vi "MAIN_HGB2_rev01.vi"() -> ()   [LabVIEW 2016]
uses:
  Producer_Case_Structure.ctl
  <vilib>/Utility/error.llb/DialogType.ctl
  <vilib>/express/express analysis/Spectral/XNode/ExpressSpectralMeasurementsBlockNode.xnode
  <vilib>/express/express analysis/Spectral/Block/exnSpectralBlock spectral measurements RMS poly.vi
  <vilib>/express/express analysis/Spectral/Block/exnSpectralBlock spectral measurements RMS array WFM.vi
  <vilib>/DAQmx/write.llb/DAQmx Write (Analog 1D DBL NChan 1Samp).vi
panel:
  out "Compressor Speed":dbl
  out "Run Loop Counter":dbl=67.0
  in  "Speed Setpoint":dbl
  in  "Operator Notes":string
  in  "Dummy Variable":dbl
  in  "Record Data":bool
  in  "Sample Rate [S/s]":dbl=10.0
  in  "file path":path=path "S:/002 - Projects/200804 AECSSB/6-Testing/TDMS Data/raw/080421-1"
  in  "Stop":bool=TRUE
  in  "Tab Control":T1(tab)=enum."Pressure & Temperature"
  out "System Temperatures":waveform(dbl)[](graph)=[{"t0"=timestamp(3710938237.209422 s since 1904-01-01), "dt"=0.1, "Y"=[25.06420596580779], "attributes"=variant("NI_ChannelName"=variant(string "T_dis"), "NI_UnitDescription"=variant(string "Deg C"))}, {"t0"=timestamp(3710938237.209422 s since 1904-01-01), "dt"=0.1, "Y"=[24.5131871952291], "attributes"=variant("NI_ChannelName"=variant(string "T_liq_mix"), "NI_UnitDescription"=variant(string "Deg C"))}, {"t0"=timestamp(3710938237.209422 s since 1904-01-01), "dt"=0.1, "Y"=[24.404692160048143], "attributes"=variant("NI_ChannelName"=variant(string "T_gas_mix"), "NI_UnitDescription"=variant(string "Deg C"))}, {"t0"=timestamp(3710938237.209422 s since 1904-01-01), "dt"=0.1, "Y"=[24.9517211018332], "attributes"=variant("NI_ChannelName"=variant(string "T_wf_cond_out"), "NI_UnitDescription"=variant(string "Deg C"))}, {"t0"=timestamp(3710938237.209422 s since 1904-01-01), "dt"=0.1, "Y"=[24.75846841874906], "attributes"=variant("NI_ChannelName"=variant(string "T_cf_in"), "NI_UnitDescription"=variant(string "Deg C"))}]
  out "Power Constituents":waveform(dbl)[](graph)=[{"t0"=timestamp(3710938237.209422 s since 1904-01-01), "dt"=0.1, "Y"=[-0.0627204059992863], "attributes"=variant("NI_ChannelName"=variant(string "Voltage"))}, {"t0"=timestamp(3710938237.209422 s since 1904-01-01), "dt"=0.1, "Y"=[-0.029340257114334634], "attributes"=variant("NI_ChannelName"=variant(string "Frequency"))}, {"t0"=timestamp(3710938237.0104485 s since 1904-01-01), "dt"=0.1, "Y"=[], "attributes"=variant("NI_ChannelName"=variant(string "Torque"))}]
  out "System Pressures":waveform(dbl)[](graph)=[{"t0"=timestamp(3710938237.209422 s since 1904-01-01), "dt"=0.1, "Y"=[653.0149804276925], "attributes"=variant("NI_ChannelName"=variant(string "P_comp_suc"))}, {"t0"=timestamp(3710938237.209422 s since 1904-01-01), "dt"=0.1, "Y"=[652.9848572024544], "attributes"=variant("NI_ChannelName"=variant(string "P_comp_dis"))}, {"t0"=timestamp(3710938237.209422 s since 1904-01-01), "dt"=0.1, "Y"=[653.0856354357659], "attributes"=variant("NI_ChannelName"=variant(string "P_comp_int"))}]
  out "Mass Flow":waveform(dbl)(graph)={"t0"=timestamp(3710938237.209422 s since 1904-01-01), "dt"=0.1, "Y"=[-2.0362630357040334e-05], "attributes"=variant("NI_ChannelName"=variant(string "m_dot_wf"))}
  out "Raw Acceleration":waveform(dbl)[](graph)
  out "Accel. Spectrum":cluster{"f0":dbl, "df":dbl, "magnitude":dbl[]}[](graph)
  in  "?":path=path "C:/Users/ASITest/Desktop/REFPROP"
  in  "Working Fluid":string="R134A.FLD"
  out "Sound":waveform(dbl)(graph)
  in  "Range":enum16{"40-70 dB", "auto", "60-90 dB"}(ring)
  in  "Ambient Noise [dB]":dbl=74.0
  # "Stop VI"
  # "Air Squared Hot Gas Bypass Test Stand"
  # "Point to where REFPROP is..."
  # "Registar Index of Calc Characteristics"
  # "INPUT NEEDED"
  # "0 = No\n1 = Yes"
  # "0 = No\n1 = Yes"
  # "UNITS:\nkg/s\nC\nRPM\nkPa\nV\nA"
  # "... where is the sensor in the initialization indexing?"
  # "Must have sound meter set up to manual range:\n1. click 'RNG' button on the meter \n2. the value displayed under 'SPL' on the display is the min of the range\n3. ensure the meter is on 'FAST' mode by clicking 'F/S', 'FAST' will be read on display\n4. use the A/C to select 'A' mode displayed on meter\n5. BEFORE INITIALIZING - set ambient noise level to whatever the sensor measures before running\n* the extech 407730 display frequency is not as high as the display freq here, so peak values\nmay not be seen on the sound meter display."
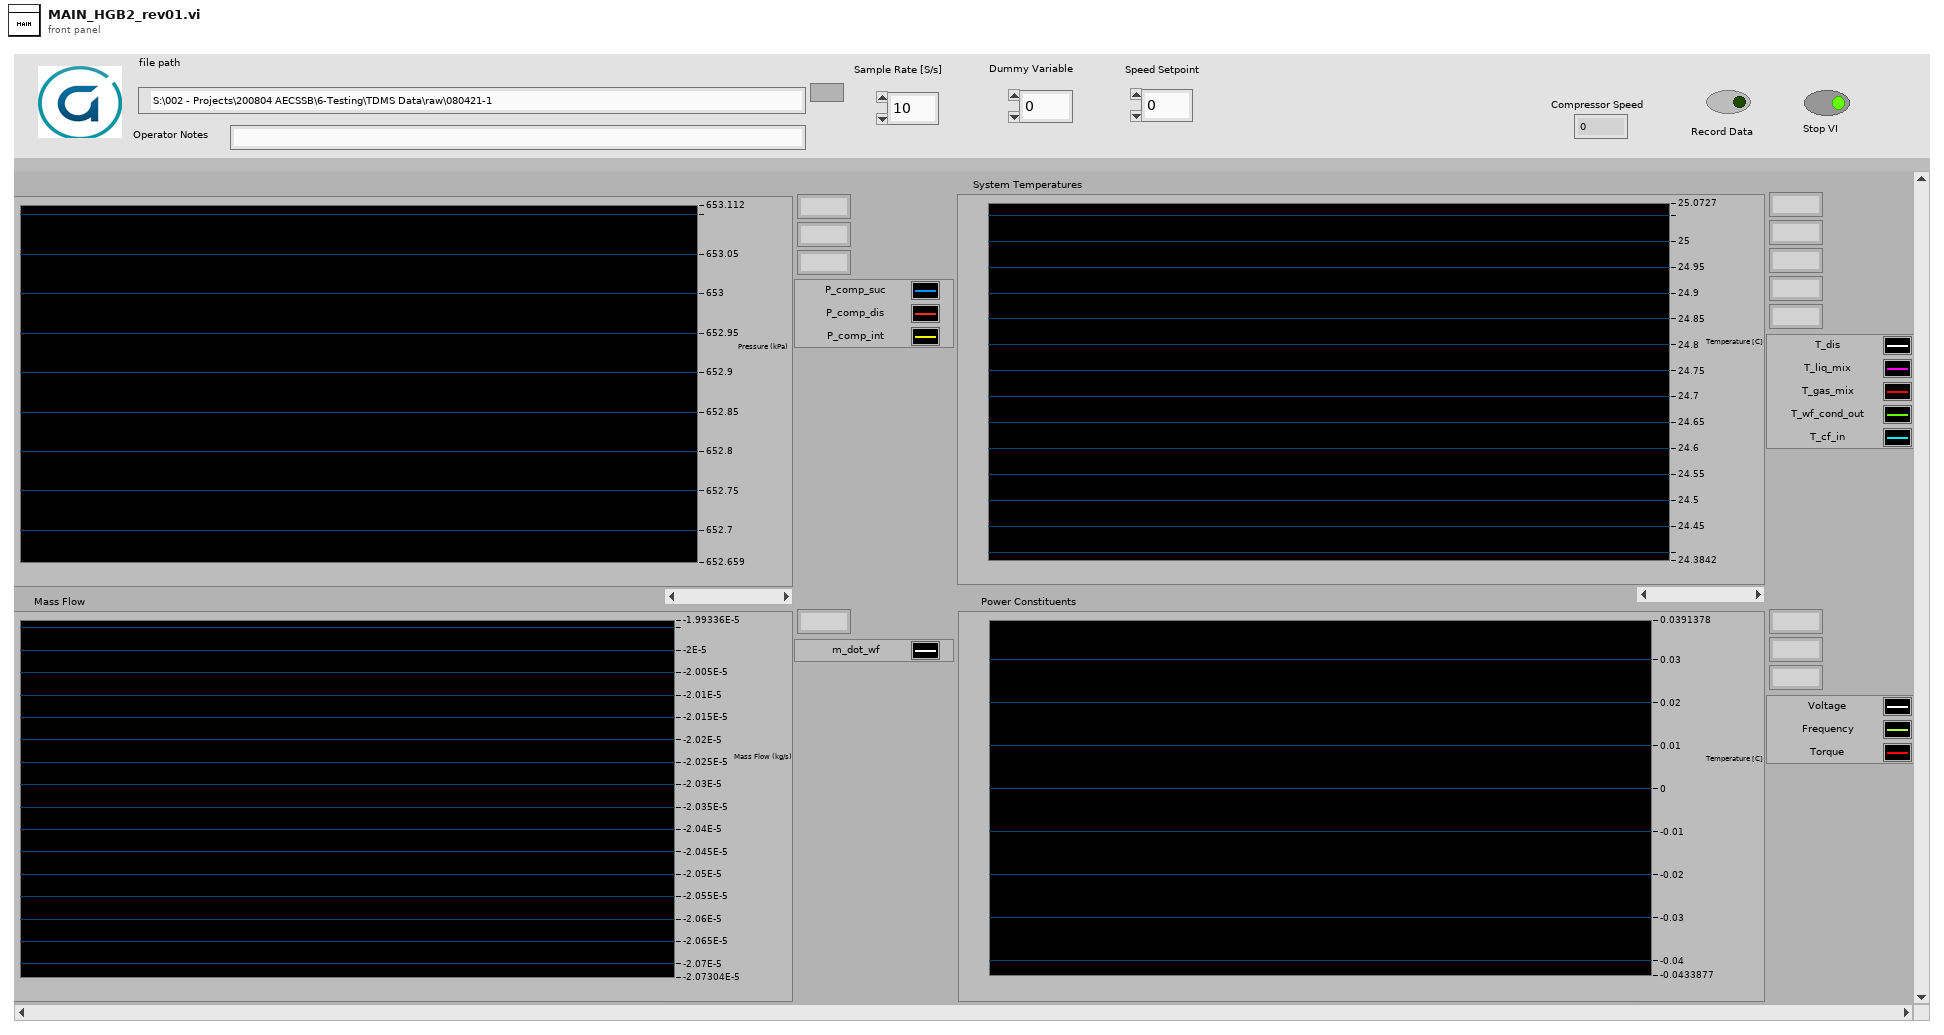
[diagram p1: front panel]
types:
  T1 = enum32{"Schematic", "Pressure & Temperature", "Power", "Acceleration", "Efficiency", "Noise"}
  T2 = typedef "Producer_Case_Structure.ctl" = enum16{"Initialize", "Read", "Write", "Display", "Queue", "Error"}
  T3 = enum16{"open", "open or create", "create or replace", "create", "open (read-only)"}
  T4 = cluster{"Data Main":waveform(dbl)[], "Accelerometer":waveform(dbl)[], "Dummy Variable":dbl, "Operator Notes":string, "RMS Current [A]":dbl, "Sound":waveform(dbl)[], "Eff. Data":waveform(dbl)[], "NI 6001":waveform(dbl)[], "Speed Setpoint":dbl}
  T5 = enum16{"System Run", "Manual", "System Off", "Defrost On", "Shutdown", "Stop"}
  T6 = typedef "DialogType.ctl" = u16
  T7 = cluster{"averaging mode":u16, "weighting mode":u16, "number of averages":u32}
  T8 = cluster{"dB On (F)":bool, "unwrap phase (F)":bool, "convert to degree (F)":bool}
  T9 = cluster{"All Channels":tag[], "All Labels":string[], "All Units":string[], "Slope":dbl[], "Y-Intercept":dbl[]}
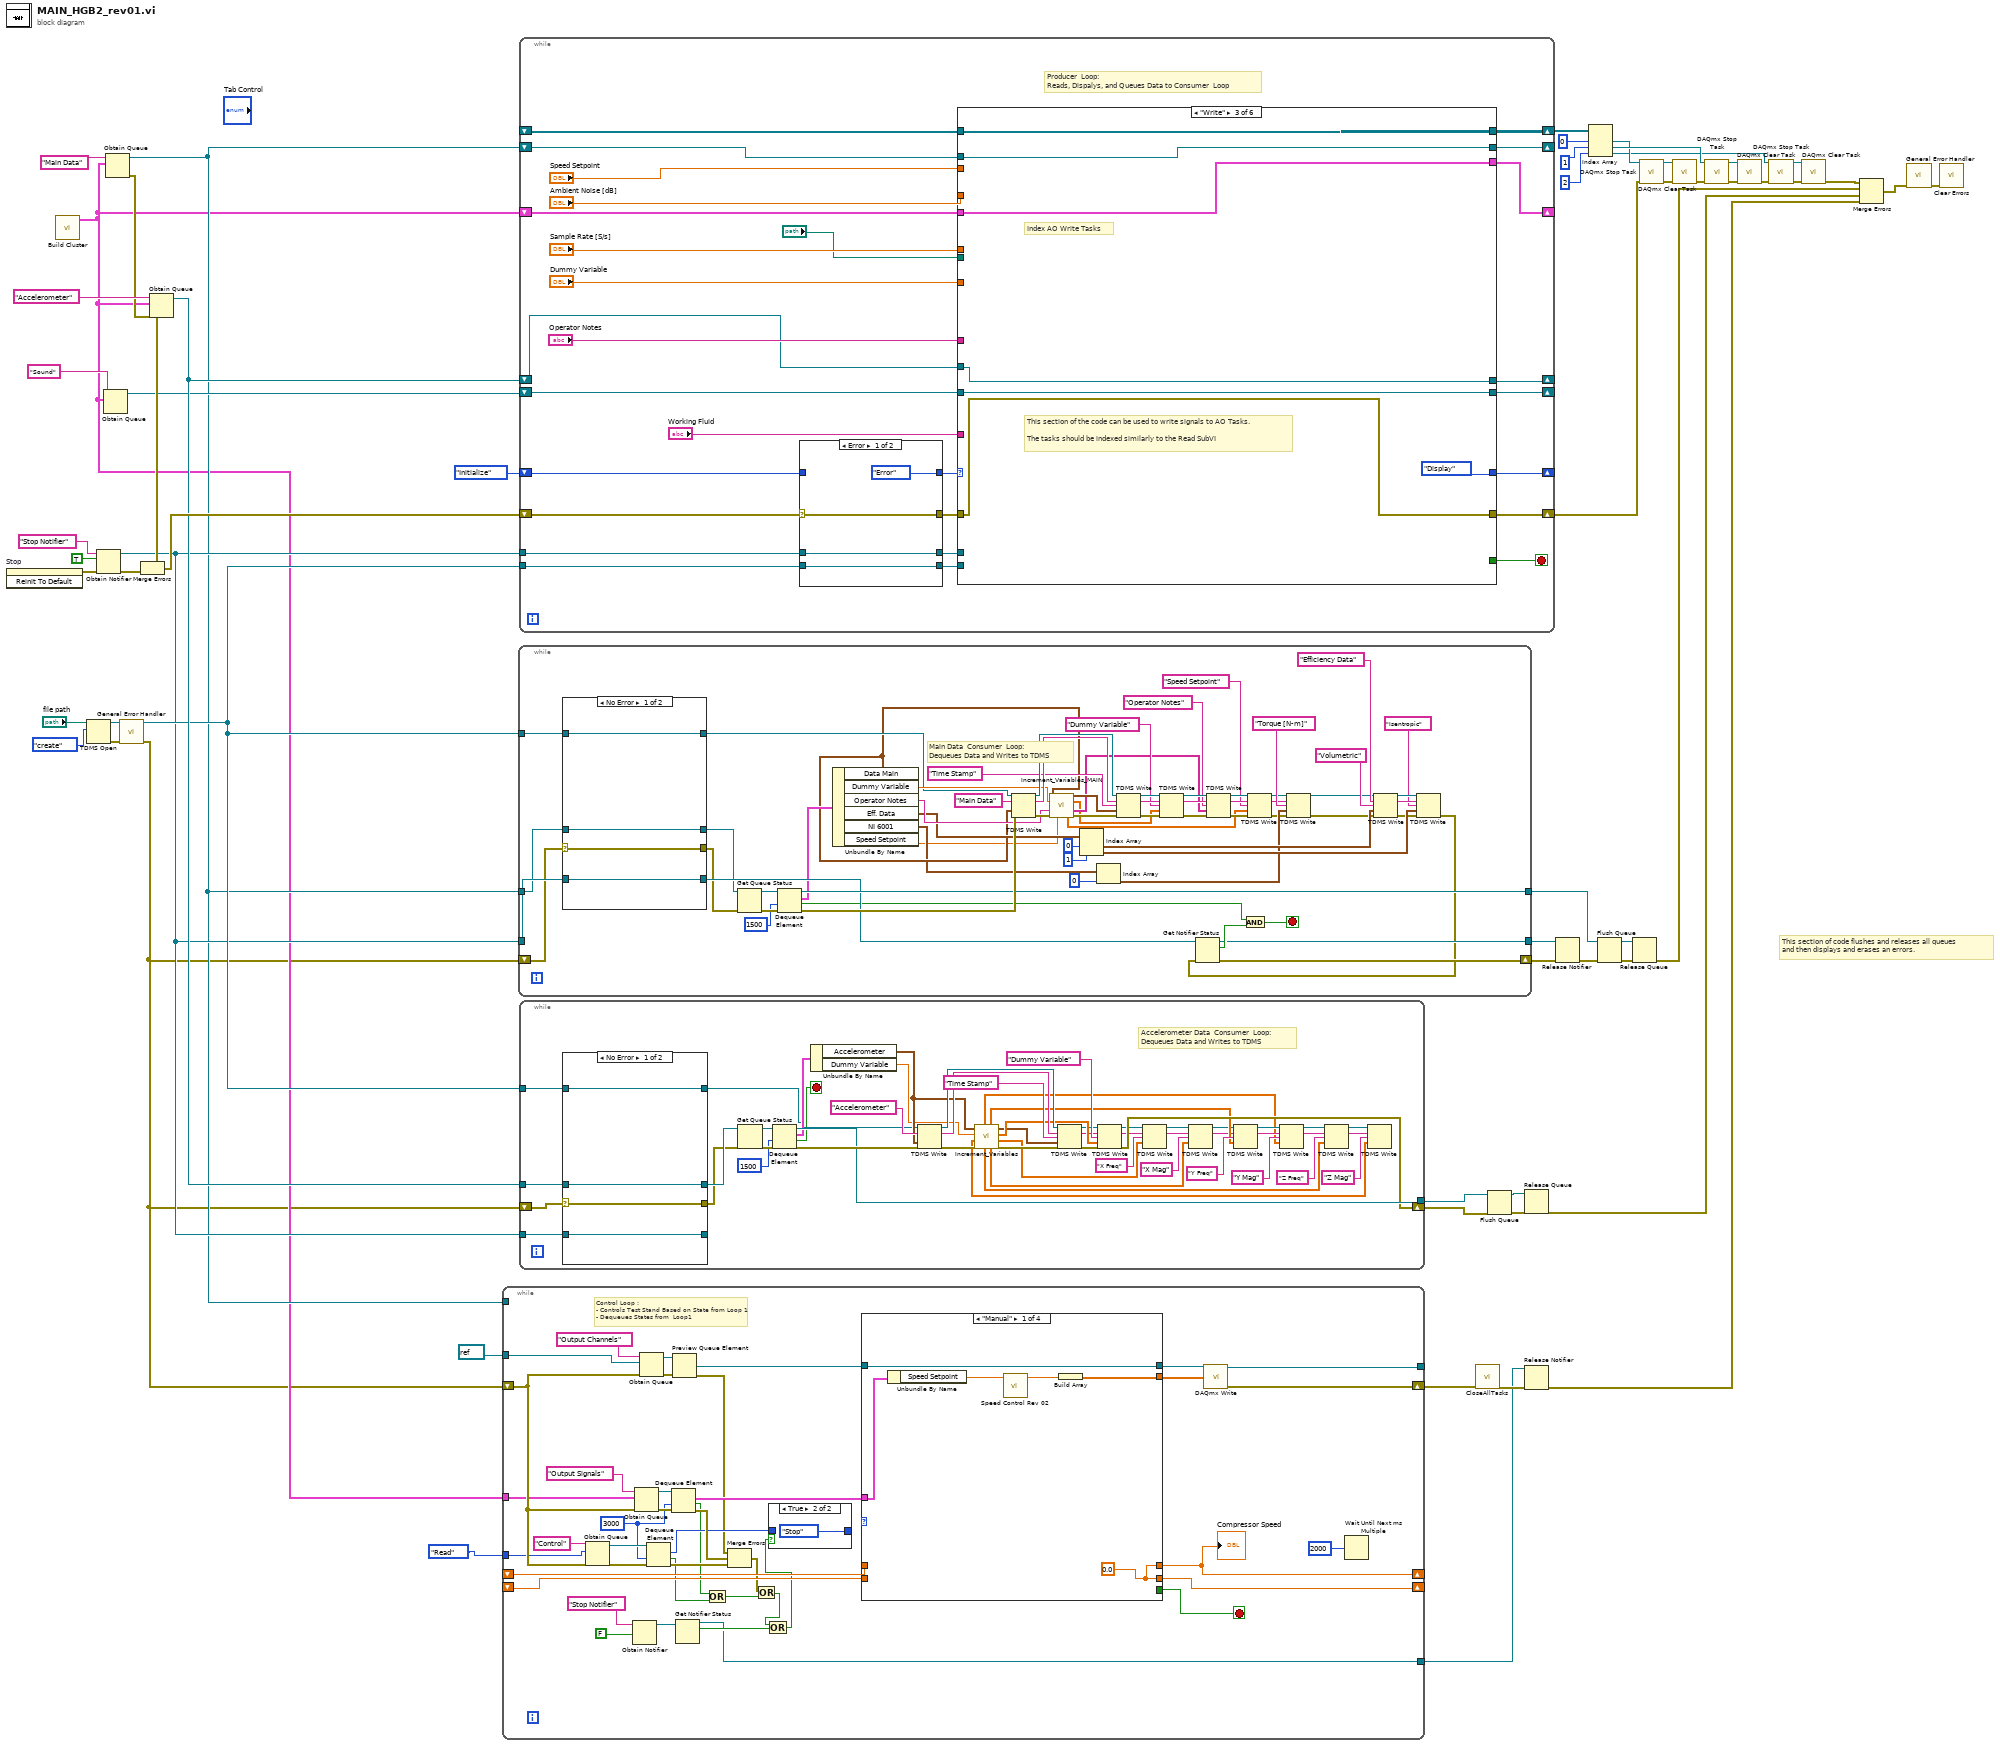
[diagram p0: block diagram]
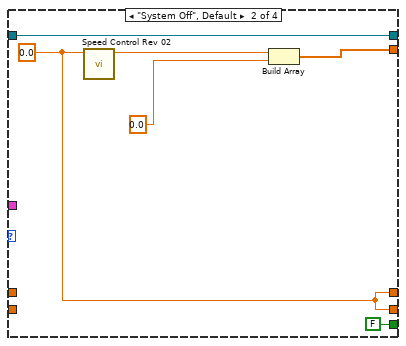
[diagram p3: hidden frame]
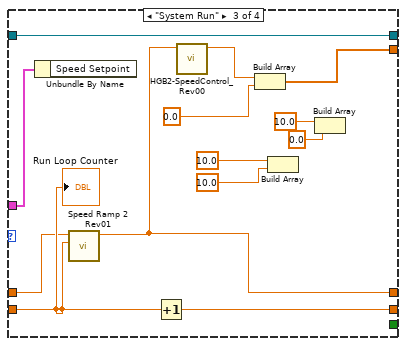
[diagram p4: hidden frame]
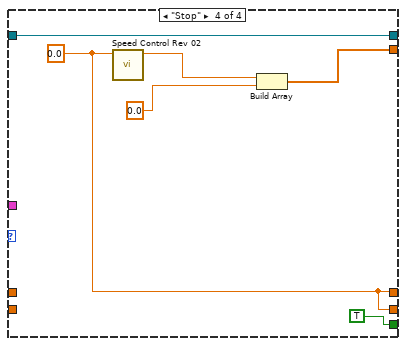
[diagram p5: hidden frame]
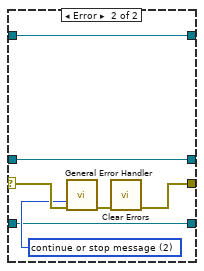
[diagram p6: hidden frame]
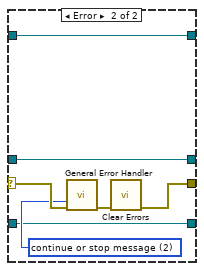
[diagram p7: hidden frame]
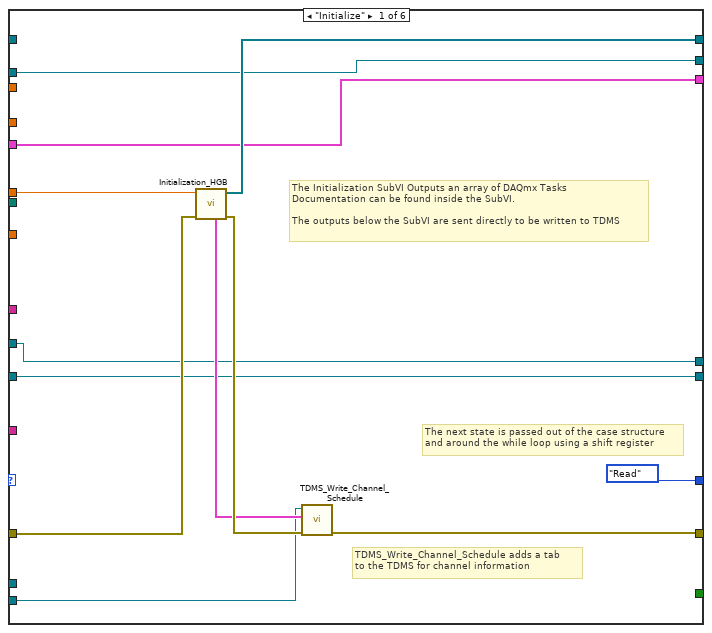
[diagram p8: hidden frame]
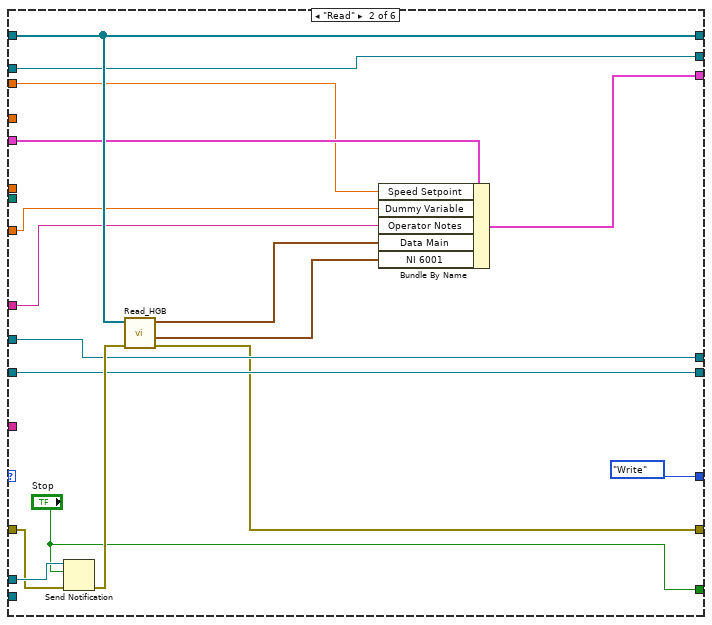
[diagram p9: hidden frame]
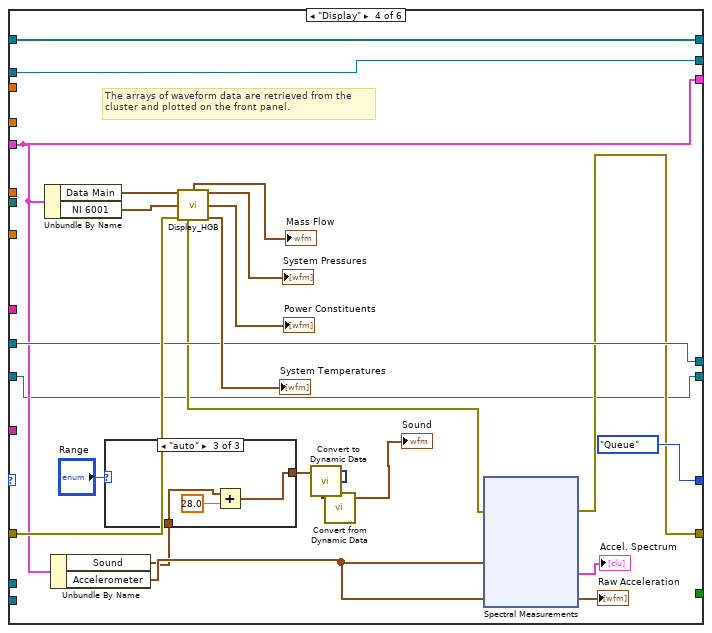
[diagram p10: hidden frame]
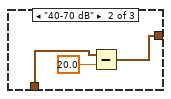
[diagram p12: hidden frame]
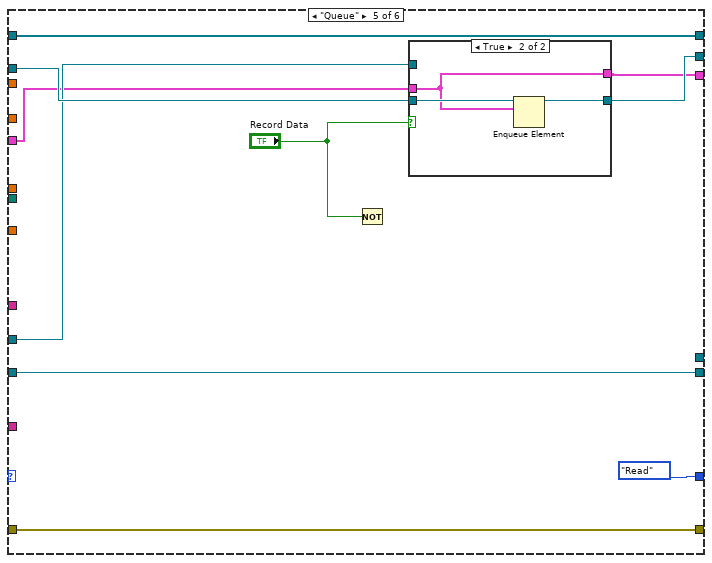
[diagram p13: hidden frame]
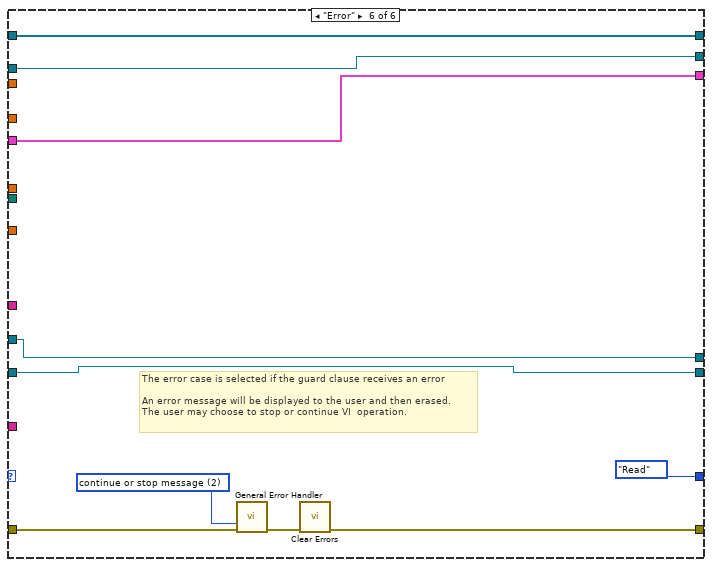
[diagram p15: hidden frame]
diagram:
  # "This section of code flushes and releases all queues \nand then displays and erases an errors."
  n1 = invoke on="Stop" class="Bool (strict)" method="Reinit To Default"() -> (error out=w52:errorcluster)  [unwired: 3 in, 2 out]
  n2 = call "Build Cluster.vi"() -> ("output cluster"=w13:T4)  [unwired: 11 in]
  n3 = TDMS Open(10:T3."create" ("operation (0:open)"), 11:"file path") -> (0:w47:errorcluster, 3:w23:refnum<k34>)  [unwired: 5 in]
  n4 = Obtain Notifier(name (unnamed)="Stop Notifier", notification data type=TRUE, error in (no error)=w52) -> (notifier out=w22:refnum<notifier>, error out=w45:errorcluster)  [unwired: 1 in, 1 out]
  n5 = Obtain Queue(name (unnamed)="Sound", element data type=w13) -> (queue out=w24:refnum<queue>)  [unwired: 3 in, 2 out]
  n6 = Obtain Queue(name (unnamed)="Main Data", element data type=w13) -> (queue out=w14:refnum<queue>, error out=w32:errorcluster)  [unwired: 3 in, 1 out]
  n7 = call <vilib>:"General Error Handler.vi"("error in (no error)"=w47) -> ("error out"=w2:errorcluster)  [unwired: 10 in, 4 out]
  n8 = Obtain Queue(name (unnamed)="Accelerometer", element data type=w13, error in (no error)=w32) -> (queue out=w30:refnum<queue>, error out=w31:errorcluster)  [unwired: 2 in, 1 out]
  n9 = Merge Errors(w31, w45) -> (w58:errorcluster)
  n10 = while {
    tunnel: [w95] -> _
    shift-right: [w63] -> w12
    shift-left: w2 -> [w79]
    tunnel: refnum<k21> refnum ("task in") -> [w87]
    shift-right: [w60] -> _
    shift-left: _ -> [w82]
    shift-right: [w61] -> _
    shift-left: _ -> [w81]
    tunnel: w14 -> [_]
    tunnel: w13 -> [w65]
    tunnel: [w64] -> w9
    tunnel: Producer_Case_Structure."Read" ("Enum") -> [w59]
    stop <- w74 stop-if-true
    w77 = 3000 ("timeout in ms (-1)")
    # "Control Loop :\n- Controls Test Stand Based on State from Loop 1\n- Dequeues States from  Loop1"
    n11 = Obtain Queue(name (unnamed)="Control", element data type=w59, error in (no error)=w79) -> (queue out=w94:refnum<queue>, error out=w80:errorcluster)  [unwired: 2 in, 1 out]
    n12 = Obtain Notifier(name (unnamed)="Stop Notifier", notification data type=FALSE) -> (notifier out=w66:refnum<notifier>)  [unwired: 2 in, 2 out]
    n13 = Obtain Queue(name (unnamed)="Output Signals", element data type=w65, error in (no error)=w79) -> (queue out=w91:refnum<queue>, error out=w85:errorcluster)  [unwired: 2 in, 1 out]
    n14 = Obtain Queue(name (unnamed)="Output Channels", element data type=w87, error in (no error)=w79) -> (queue out=w88:refnum<queue>, error out=w86:errorcluster)  [unwired: 2 in, 1 out]
    n15 = Dequeue Element(queue=w94, timeout in ms (-1)=w77, error in (no error)=w80) -> (element=w78:T2, timed out?=w75:bool, error out=w83:errorcluster)  [unwired: 1 out]
    n16 = Dequeue Element(queue=w91, timeout in ms (-1)=w77, error in (no error)=w85) -> (element=w90:T4, timed out?=w76:bool, error out=w84:errorcluster)  [unwired: 1 out]
    n17 = Preview Queue Element(queue=w88, error in (no error)=w86) -> (element=w89:refnum<k21>, error out=w62:errorcluster)  [unwired: 1 in, 2 out]
    n18 = Get Notifier Status(notifier=w66) -> (notifier out=w64:refnum<notifier>, current notification=w71:bool)  [unwired: 1 in, 3 out]
    n19 = Or(x=w76, y=w75) -> (x .or. y?=w73:bool)
    n20 = Merge Errors(w62, w84, w83) -> (w72:errorcluster)
    n21 = Or(x=w72, y=w73) -> (x .or. y?=w70:bool)
    n22 = Or(x=w70, y=w71) -> (x .or. y?=w69:bool)
    n23 = case shown="True" w69 {
      tunnel: w78 -> [w100 _]
      tunnel: [w100 T5."Stop"] -> _
      frame False {
      }
      frame True {
      }
    }
    n24 = case shown="\"Manual\"" {
      selector: _ -> [_ _ _ _]
      tunnel: [_ FALSE ("stop") _ TRUE ("stop")] -> w74
      tunnel: w89 -> [w106 w111 w126 w134]
      tunnel: [w105 w112 w127 w132] -> w97
      tunnel: [w106 w111 w126 w134] -> w96
      tunnel: w90 -> [w103 _ w125 _]
      tunnel: [w104 w109 w119 w129] -> w60
      tunnel: w82 -> [_ _ w117 _]
      tunnel: [w104 w109 w116 w129] -> w61
      tunnel: w81 -> [_ _ w115 _]
      frame "Manual" {
        w104 = 0.0 ("Speed Setpoint 2")
        n25 = Unbundle By Name(w103) -> ("Speed Setpoint"=w102:dbl)
        n26 = call "Speed Control Rev 02.vi"("Set Speed"=w102) -> ("Speed Control Output"=w107:dbl)  [unwired: 10 in]
        n27 = Build Array(w107) -> (w105:dbl[])
      }
      frame "System Off", Default {
        w109 = 0.0 ("Speed Setpoint 2")
        n28 = call "Speed Control Rev 02.vi"("Set Speed"=w109) -> ("Speed Control Output"=w113:dbl)  [unwired: 10 in]
        n29 = Build Array(w113, 0.0 ("Speed Setpoint 2")) -> (w112:dbl[])
      }
      frame "System Run" {
        n30 = Unbundle By Name(w125) -> ()  [unwired: 1 out]
        n31 = call "Speed Ramp 2 Rev01.vi"("Counter"=w117, "Compressor Speed In"=w115) -> ("Compressor Speed Out"=w116:dbl)  [unwired: 8 in, 1 out]
        n32 = Increment(x=w117) -> (x+1=w119:dbl)
        n33 = call "HGB2-SpeedControl_Rev00.vi"("Set Speed"=w116) -> ("Speed Control Output"=w128:dbl)  [unwired: 10 in]
        n34 = Build Array(w128, 0.0 ("Speed Setpoint 2")) -> (w127:dbl[])
        n35 = Build Array(10.0 ("Speed Setpoint 2"), 10.0 ("Speed Setpoint 2")) -> (w122:dbl[])
        n36 = Build Array(10.0 ("Speed Setpoint 2"), 0.0 ("element")) -> (w120:dbl[])
        "Run Loop Counter" <- w117
      }
      frame "Stop" {
        w129 = 0.0 ("Speed Setpoint 2")
        n37 = call "Speed Control Rev 02.vi"("Set Speed"=w129) -> ("Speed Control Output"=w133:dbl)  [unwired: 10 in]
        n38 = Build Array(w133, 0.0 ("Speed Setpoint 2")) -> (w132:dbl[])
      }
    }
    "Compressor Speed" <- w61
    n39 = call-poly <vilib>:"DAQmx Write.vi"("task/channels in"=w96, "data"=w97) -> ("task out"=w95:refnum<k21>, "error out"=w63:errorcluster)  [unwired: 11 in, 1 out]
    n40 = Wait Until Next ms Multiple(millisecond multiple=u32 2000) -> ()  [unwired: 1 out]
  }
  n41 = while {
    tunnel: w23 -> [w188]
    tunnel: [w198] -> w43
    tunnel: w14 -> [w189]
    tunnel: w22 -> [w191]
    shift-right: [w196] -> w41
    shift-left: w2 -> [w187]
    tunnel: [w166] -> w39
    stop <- w193 stop-if-true
    # "Main Data  Consumer  Loop: \nDequeues Data and Writes to TDMS"
    n42 = case shown="No Error" w187 {
      selector: w187 -> [w204 w210]
      tunnel: [w204 w209] -> w169
      tunnel: w191 -> [w203 w205]
      tunnel: [w203 w205] -> w192
      tunnel: [w202 w207] -> w190
      tunnel: w189 -> [w202 w207]
      tunnel: [w201 w206] -> w167
      tunnel: w188 -> [w201 w206]
      frame No Error {
      }
      frame Error {
        w208 = T6 2 items=["no dialog", "OK message", "continue or stop message", "OK message + warnings", "continue/stop + warnings"] ("type of dialog (OK msg:1)")
        n43 = call <vilib>:"General Error Handler.vi"("type of dialog (OK msg:1)"=w208, "error in (no error)"=w210) -> ("error out"=w211:errorcluster)  [unwired: 9 in, 4 out]
        n44 = call <vilib>:"Clear Errors.vi"("error in (no error)"=w211) -> ("error out"=w209:errorcluster)  [unwired: 5 in, 1 out]
      }
    }
    n45 = Get Queue Status(queue=w190, error in (no error)=w169) -> (queue out=w195:refnum<queue>, error out=w199:errorcluster)  [unwired: 1 in, 6 out]
    n46 = Dequeue Element(queue=w195, timeout in ms (-1)=1500, error in (no error)=w199) -> (queue out=w198:refnum<queue>, element=w168:T4, timed out?=w186:bool, error out=w200:errorcluster)
    n47 = Unbundle By Name(w168) -> ("Data Main"=w147:waveform(dbl)[], "Dummy Variable"=w176:dbl, "Operator Notes"=w164:string, "Eff. Data"=w148:waveform(dbl)[], "NI 6001"=w145:waveform(dbl)[], "Speed Setpoint"=w136:dbl)
    n48 = TDMS Write(0:w167, 5:"Main Data" ("group name in (Untitled)"), 9:w147, 11:w200) -> (4:w183:refnum<k34>, 6:w181:string, 15:w184:errorcluster)  [unwired: 2 in, 1 out]
    n49 = call "Increment_Variables_MAIN.vi"("Data Main"=w147, "Dummy Variable"=w176, "Operator Notes"=w164, "error in 2"=w184, "Speed Setpoint"=w136) -> ("Time Stamp"=w177:timestamp[], "Dummy Variable Array"=w135:dbl[], "Operator Notes Array"=w165:string[], "Speed Setpoint Array"=w160:dbl[], "error IO"=w185:errorcluster)  [unwired: 6 in]
    n50 = Index Array(array=w148, index #1=0 ("index"), index #2=1 ("index")) -> (element #1=w156:waveform(dbl), element #2=w153:waveform(dbl))
    n51 = Index Array(array=w145, index=0) -> (element=w141:waveform(dbl))
    n52 = TDMS Write(0:w183, 5:w181, 7:"Time Stamp" ("group name in (Untitled)"), 9:w177, 11:w185) -> (4:w180:refnum<k34>, 6:w178:string, 15:w179:errorcluster)  [unwired: 1 in, 1 out]
    n53 = TDMS Write(0:w180, 5:w178, 7:"Dummy Variable" ("group name in (Untitled)"), 9:w135, 11:w179) -> (4:w174:refnum<k34>, 6:w173:string, 15:w175:errorcluster)  [unwired: 1 in, 1 out]
    n54 = TDMS Write(0:w174, 5:w173, 7:"Operator Notes" ("group name in (Untitled)"), 9:w165, 11:w175) -> (4:w161:refnum<k34>, 6:w162:string, 15:w163:errorcluster)  [unwired: 1 in, 1 out]
    n55 = TDMS Write(0:w161, 5:w162, 7:"Speed Setpoint" ("group name in (Untitled)"), 9:w160, 11:w163) -> (4:w143:refnum<k34>, 6:w142:string, 15:w140:errorcluster)  [unwired: 1 in, 1 out]
    n56 = TDMS Write(0:w143, 5:w142, 7:"Torque [N-m]" ("channel name(s) in (Untitled)"), 9:w141, 11:w140) -> (4:w139:refnum<k34>, 15:w138:errorcluster)  [unwired: 1 in, 2 out]
    n57 = TDMS Write(0:w139, 5:"Efficiency Data" ("group name in (Untitled)"), 7:"Volumetric" ("channel name(s) in (Untitled)"), 9:w156, 11:w138) -> (4:w152:refnum<k34>, 6:w151:string, 15:w149:errorcluster)  [unwired: 1 in, 1 out]
    n58 = TDMS Write(0:w152, 5:w151, 7:"Isentropic" ("channel name(s) in (Untitled)"), 9:w153, 11:w149) -> (15:w137:errorcluster)  [unwired: 1 in, 3 out]
    n59 = Get Notifier Status(notifier=w192, error in (no error)=w137) -> (notifier out=w166:refnum<notifier>, current notification=w197:bool, error out=w196:errorcluster)  [unwired: 2 out]
    n60 = And(x=w186, y=w197) -> (x .and. y?=w193:bool)
  }
  n61 = while {
    shift-right: [w232] -> _
    shift-left: Producer_Case_Structure."Initialize" ("Enum") -> [w238]
    shift-right: [w234] -> w49
    shift-left: _ -> [w233]
    tunnel: w22 -> [w239]
    shift-right: [w229] -> _
    shift-left: w13 -> [w228]
    shift-right: [w226] -> _
    shift-left: w14 -> [w225]
    shift-right: [w235] -> w8
    shift-left: w58 -> [w227]
    tunnel: w23 -> [w220]
    shift-right: [w218] -> _
    shift-left: w30 -> [w219]
    shift-right: [w217] -> _
    shift-left: w24 -> [w216]
    stop <- w231 stop-if-true
    # "Producer  Loop: \nReads, Dispalys, and Queues Data to Consumer  Loop"
    n62 = case shown="Error" w227 {
      selector: w227 -> [w341 w347]
      tunnel: [w341 w347] -> w236
      tunnel: w239 -> [w343 w346]
      tunnel: [w343 w346] -> w230
      tunnel: w238 -> [_ w345]
      tunnel: [Producer_Case_Structure."Error" ("Enum") w345] -> w237
      tunnel: [w340 w344] -> w221
      tunnel: w220 -> [w340 w344]
      frame Error {
      }
      frame No Error {
      }
    }
    n63 = case shown="\"Write\"" w237 {
      tunnel: w236 -> [w251 w263 w270 w297 w322 w336]
      tunnel: [w244 w253 w270 w289 w322 w333] -> w235
      tunnel: [w250 w264 w275 w295 w323 w337] -> w234
      tunnel: w233 -> [_ w264 w275 w295 w323 w337]
      tunnel: [Producer_Case_Structure."Read" ("Enum") Producer_Case_Structure."Write" ("Enum") Producer_Case_Structure."Display" ("Enum") Producer_Case_Structure."Queue" ("Enum") Producer_Case_Structure."Read" ("Enum") Producer_Case_Structure."Read" ("Enum")] -> w232
      tunnel: [_ "Stop" _ _ _ _] -> w231
      tunnel: w230 -> [_ w266 _ _ _ _]
      tunnel: [w246 w261 w273 w288 w319 w335] -> w229
      tunnel: w228 -> [w246 w256 w273 w288 w317 w335]
      tunnel: [w248 w262 w272 w293 w320 w332] -> w226
      tunnel: w225 -> [w248 w262 w272 w293 w321 w332]
      tunnel: "Sample Rate [S/s]" -> [w247 _ _ _ _ _]
      tunnel: "Dummy Variable" -> [_ w258 _ _ _ _]
      tunnel: "Operator Notes" -> [_ w260 _ _ _ _]
      tunnel: w221 -> [w242 _ _ _ _ _]
      tunnel: w219 -> [w241 w259 w271 w291 w318 w331]
      tunnel: [w241 w259 w271 w291 _ w331] -> w218
      tunnel: [w240 w257 w269 w286 w316 w330] -> w217
      tunnel: w216 -> [w240 w257 w269 w286 w316 w330]
      tunnel: "Ambient Noise [dB]" -> [_ _ _ _ _ _]
      tunnel: "?" -> [_ _ _ _ _ _]
      tunnel: "Working Fluid" -> [_ _ _ _ _ _]
      tunnel: "Speed Setpoint" -> [_ w254 _ _ _ _]
      frame "Initialize" {
        # "TDMS_Write_Channel_Schedule adds a tab \nto the TDMS for channel information"
        # "The next state is passed out of the case structure \nand around the while loop using a shift register"
        # "The Initialization SubVI Outputs an array of DAQmx Tasks\nDocumentation can be found inside the SubVI.\n\nThe outputs below the SubVI are sent directly to be written to TDMS"
        n64 = call "Initialization_HGB.vi"("error in"=w251, "Sample Rate"=w247) -> ("error out"=w245:errorcluster, "Task Array"=w250:refnum<k21>[], "output cluster"=w243:T9)  [unwired: 7 in]
        n65 = call "TDMS_Write_Channel_Schedule.vi"("error in (no error)"=w245, "output cluster"=w243, "Refnum in"=w242) -> ("error out"=w244:errorcluster)  [unwired: 8 in]
      }
      frame "Read" {
        n66 = Send Notification(notification="Stop", notifier=w266, error in (no error)=w263) -> (error out=w268:errorcluster)  [unwired: 1 out]
        n67 = call "Read_HGB.vi"("error in (no error)"=w268, "Task Array"=w264) -> ("error out"=w253:errorcluster, "NI 6001"=w252:waveform(dbl)[], "Data Main"=w255:waveform(dbl)[])  [unwired: 7 in]
        n68 = Bundle By Name(cluster=w256, "Speed Setpoint"=w254, "Dummy Variable"=w258, "Operator Notes"=w260, "Data Main"=w255, "NI 6001"=w252) -> (w261:T4)
      }
      frame "Write" {
        # "This section of the code can be used to write signals to AO Tasks.\n\nThe tasks should be indexed similarly to the Read SubVI"
        # "Index AO Write Tasks"
      }
      frame "Display" {
        # "The arrays of waveform data are retrieved from the \ncluster and plotted on the front panel."
        n69 = Unbundle By Name(w288) -> ("Data Main"=w280:waveform(dbl)[], "NI 6001"=w276:waveform(dbl)[])
        n70 = Unbundle By Name(w288) -> ("Sound"=w285:waveform(dbl)[], "Accelerometer"=w287:waveform(dbl)[])
        "Raw Acceleration" <- w287
        n71 = case shown="\"auto\"" "Range" {
          tunnel: [w298 w299 w302] -> w283
          tunnel: w285 -> [w298 w300 w303]
          frame "60-90 dB" {
          }
          frame "40-70 dB" {
            n72 = Subtract(x=w300, y=20.0) -> (x-y=w299:waveform(dbl)[])
          }
          frame "auto" {
            n73 = Add(x=w303, y=28.0) -> (x+y=w302:waveform(dbl)[])
          }
        }
        n74 = call "Display_HGB.vi"("data"=w280, "NI 6001"=w276, "error in (no error)"=w297) -> ("Mass Flow"=→"Mass Flow":waveform(dbl), "System Pressures"=→"System Pressures":waveform(dbl)[], "Power Constituents"=→"Power Constituents":waveform(dbl)[], "error out"=w290:errorcluster, "System Temperatures"=→"System Temperatures":waveform(dbl)[])  [unwired: 8 in]
        n75 = call "Convert to Dynamic Data"("Array of Waveforms"=w283) -> ("Dynamic Data Type"=w281:dynamicdata)  [unwired: 3 in]
        n76 = call "Convert from Dynamic Data"("Dynamic Data Type"=w281) -> ("Waveform"=→"Sound":waveform(dbl))  [unwired: 3 in]
        n77 = xnode "Spectral Measurements"("Signals"=w287, "error in (no error)"=w290) -> ("FFT - (RMS)"=→"Accel. Spectrum":cluster{"f0":dbl, "df":dbl, "magnitude":dbl[]}[], "error out"=w289:errorcluster)  [unwired: 1 out]
      }
      frame "Queue" {
        n78 = Not(x="Record Data") -> ()  [unwired: 1 out]
        n79 = case shown="True" "Record Data" {
          tunnel: w317 -> [w325 w327]
          tunnel: w321 -> [w326 w328]
          tunnel: [w326 w329] -> w320
          tunnel: [w325 w327] -> w319
          tunnel: w318 -> [_ _]
          frame False {
          }
          frame True {
            n80 = Enqueue Element(queue=w328, element=w327) -> (queue out=w329:refnum<queue>)  [unwired: 2 in, 2 out]
          }
        }
      }
      frame "Error" {
        w338 = T6 2 items=["no dialog", "OK message", "continue or stop message", "OK message + warnings", "continue/stop + warnings"] ("type of dialog (OK msg:1)")
        # "The error case is selected if the guard clause receives an error\n\nAn error message will be displayed to the user and then erased. \nThe user may choose to stop or continue VI  operation."
        n81 = call <vilib>:"General Error Handler.vi"("type of dialog (OK msg:1)"=w338, "error in (no error)"=w336) -> ("error out"=w334:errorcluster)  [unwired: 9 in, 4 out]
        n82 = call <vilib>:"Clear Errors.vi"("error in (no error)"=w334) -> ("error out"=w333:errorcluster)  [unwired: 5 in, 1 out]
      }
    }
  }
  n83 = while {
    tunnel: w23 -> [w392]
    tunnel: [w398] -> w27
    tunnel: w30 -> [w393]
    tunnel: w22 -> [w395]
    shift-right: [w373] -> w21
    shift-left: w2 -> [w391]
    stop <- w372 stop-if-true
    # "Accelerometer Data  Consumer  Loop: \nDequeues Data and Writes to TDMS"
    n84 = case shown="No Error" w391 {
      selector: w391 -> [w404 w410]
      tunnel: [w404 w409] -> w383
      tunnel: w395 -> [w403 w405]
      tunnel: [w403 w405] -> _
      tunnel: [w402 w407] -> w394
      tunnel: w393 -> [w402 w407]
      tunnel: [w401 w406] -> w381
      tunnel: w392 -> [w401 w406]
      frame No Error {
      }
      frame Error {
        w408 = T6 2 items=["no dialog", "OK message", "continue or stop message", "OK message + warnings", "continue/stop + warnings"] ("type of dialog (OK msg:1)")
        n85 = call <vilib>:"General Error Handler.vi"("type of dialog (OK msg:1)"=w408, "error in (no error)"=w410) -> ("error out"=w411:errorcluster)  [unwired: 9 in, 4 out]
        n86 = call <vilib>:"Clear Errors.vi"("error in (no error)"=w411) -> ("error out"=w409:errorcluster)  [unwired: 5 in, 1 out]
      }
    }
    n87 = Get Queue Status(queue=w394, error in (no error)=w383) -> (queue out=w397:refnum<queue>, error out=w399:errorcluster)  [unwired: 1 in, 6 out]
    n88 = Dequeue Element(queue=w397, timeout in ms (-1)=1500, error in (no error)=w399) -> (queue out=w398:refnum<queue>, element=w382:T4, timed out?=w372:bool, error out=w400:errorcluster)
    n89 = Unbundle By Name(w382) -> ("Accelerometer"=w385:waveform(dbl)[], "Dummy Variable"=w380:dbl)
    n90 = TDMS Write(0:w381, 5:"Accelerometer" ("group name in (Untitled)"), 9:w385, 11:w400) -> (4:w388:refnum<k34>, 6:w386:string, 15:w389:errorcluster)  [unwired: 2 in, 1 out]
    n91 = call "Increment_Variables.vi"("error in 2"=w389, "Dummy Variable"=w380, "Accelerometer"=w385) -> ("error IO"=w390:errorcluster, "X Accel Freq Array"=w369:dbl[], "Dummy Variable Array"=w378:dbl[], "Time Stamp"=w374:timestamp[], "X Accel Mag Array"=w367:dbl[], "Y Accel Freq Array"=w350:dbl[], "Z Accel Freq Array"=w352:dbl[], "Y Accel Mag Array"=w351:dbl[], "Z Accel Mag Array"=w353:dbl[])
    n92 = TDMS Write(0:w388, 5:w386, 7:"Time Stamp" ("group name in (Untitled)"), 9:w374, 11:w390) -> (4:w375:refnum<k34>, 6:w376:string, 15:w379:errorcluster)  [unwired: 1 in, 1 out]
    n93 = TDMS Write(0:w375, 5:w376, 7:"Dummy Variable" ("group name in (Untitled)"), 9:w378, 11:w379) -> (4:w370:refnum<k34>, 6:w371:string, 15:w373:errorcluster)  [unwired: 1 in, 1 out]
    n94 = TDMS Write(0:w370, 5:w371, 7:"X Freq" ("group name in (Untitled)"), 9:w369) -> (4:w364:refnum<k34>, 6:w365:string)  [unwired: 2 in, 2 out]
    n95 = TDMS Write(0:w364, 5:w365, 7:"X Mag" ("group name in (Untitled)"), 9:w367) -> (4:w349:refnum<k34>, 6:w348:string)  [unwired: 2 in, 2 out]
    n96 = TDMS Write(0:w349, 5:w348, 7:"Y Freq" ("group name in (Untitled)"), 9:w350) -> (4:w361:refnum<k34>, 6:w360:string)  [unwired: 2 in, 2 out]
    n97 = TDMS Write(0:w361, 5:w360, 7:"Y Mag" ("group name in (Untitled)"), 9:w351) -> (4:w362:refnum<k34>, 6:w363:string)  [unwired: 2 in, 2 out]
    n98 = TDMS Write(0:w362, 5:w363, 7:"Z Freq" ("group name in (Untitled)"), 9:w352) -> (4:w359:refnum<k34>, 6:w358:string)  [unwired: 2 in, 2 out]
    n99 = TDMS Write(0:w359, 5:w358, 7:"Z Mag" ("group name in (Untitled)"), 9:w353) -> ()  [unwired: 2 in, 4 out]
  }
  n100 = call "CloseAllTasks.vi"("error in (no error)"=w12) -> ("error out"=w11:errorcluster)  [unwired: 9 in]
  n101 = Flush Queue(queue=w27, error in (no error)=w21) -> (queue out=w29:refnum<queue>, error out=w28:errorcluster)  [unwired: 1 out]
  n102 = Release Queue(queue=w29, error in (no error)=w28) -> (error out=w4:errorcluster)  [unwired: 1 in, 2 out]
  n103 = Release Notifier(notifier=w9, error in (no error)=w11) -> (error out=w3:errorcluster)  [unwired: 1 in, 2 out]
  n104 = Release Notifier(notifier=w39, error in (no error)=w41) -> (error out=w40:errorcluster)  [unwired: 1 in, 2 out]
  n105 = Index Array(array=w49, index #1=0 ("index"), index #2=1 ("index"), index #3=2 ("index")) -> (element #1=w19:refnum<k21>, element #2=w36:refnum<k21>, element #3=w15:refnum<k21>)
  n106 = Flush Queue(queue=w43, error in (no error)=w40) -> (queue out=w44:refnum<queue>, error out=w42:errorcluster)  [unwired: 1 out]
  n107 = Release Queue(queue=w44, error in (no error)=w42) -> (error out=w5:errorcluster)  [unwired: 1 in, 2 out]
  n108 = call <vilib>:"DAQmx Stop Task.vi"("task/channels in"=w19, "error in"=w8) -> ("task out"=w50:refnum<k21>, "error out"=w51:errorcluster)  [unwired: 12 in]
  n109 = call <vilib>:"DAQmx Clear Task.vi"("task in"=w50, "error in"=w51) -> ("error out"=w37:errorcluster)  [unwired: 13 in]
  n110 = call <vilib>:"DAQmx Stop Task.vi"("task/channels in"=w36, "error in"=w37) -> ("task out"=w34:refnum<k21>, "error out"=w38:errorcluster)  [unwired: 12 in]
  n111 = call <vilib>:"DAQmx Clear Task.vi"("task in"=w34, "error in"=w38) -> ("error out"=w16:errorcluster)  [unwired: 13 in]
  n112 = call <vilib>:"DAQmx Stop Task.vi"("task/channels in"=w15, "error in"=w16) -> ("task out"=w17:refnum<k21>, "error out"=w18:errorcluster)  [unwired: 12 in]
  n113 = call <vilib>:"DAQmx Clear Task.vi"("task in"=w17, "error in"=w18) -> ("error out"=w7:errorcluster)  [unwired: 13 in]
  n114 = Merge Errors(w7, w5, w4, w3) -> (w6:errorcluster)
  n115 = call <vilib>:"General Error Handler.vi"("error in (no error)"=w6) -> ("error out"=w25:errorcluster)  [unwired: 10 in, 4 out]
  n116 = call <vilib>:"Clear Errors.vi"("error in (no error)"=w25) -> ()  [unwired: 5 in, 2 out]
